vi "dfd_FIR Linear Phase Validation.vi"(8 "error in (no error)":errorcluster, 11 "H(n) in":dbl[](array[numeric])) -> (0 "error out":errorcluster, 3 "H(n) out":dbl[](array[numeric]))   [LabVIEW 2017, in "NI_DigFilter_Design.lvlib"]
uses:
  <vilib>/addons/Digital Filter Design/NI_DigFilter_Design.lvlib
  <vilib>/addons/Digital Filter Design/_Misc.llb/dfd_X Equal Y (Array).vi
  <vilib>/addons/Digital Filter Design/_Misc.llb/dfd_Error Handlers (Single).vi
  <vilib>/addons/Digital Filter Design/NI_DigFilterLicensed.lvlib
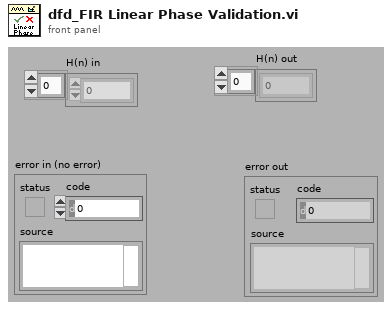
[diagram p1: front panel]
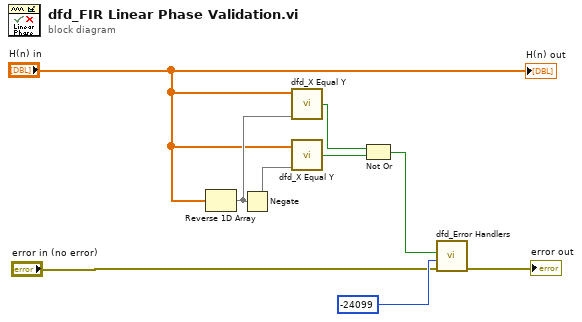
[diagram p0: block diagram]
diagram:
  n1 = Reverse 1D Array(array="H(n) in") -> (reversed array=w5:dbl[])
  n2 = Negate(x=w5) -> (-x=w3:dbl[])
  n3 = call-poly <vilib>:"dfd_X Equal Y.vi"("x"="H(n) in", "y"=w5) -> ("x = y?"=w1:bool)  [unwired: 1 in, 4 out]
  n4 = call-poly <vilib>:"dfd_X Equal Y.vi"("x"="H(n) in", "y"=w3) -> ("x = y?"=w2:bool)  [unwired: 1 in, 4 out]
  n5 = Not Or(1:w2, 2:w1) -> (0:w6:bool)
  n6 = call-poly <vilib>:"dfd_Error Handlers.vi"("error in (no error)"="error in (no error)", "error code"=-24099 ("ERR_NOT_LINEAR_PHASE_FIR"), "condition failed?"=w6) -> ("error out"=→"error out":errorcluster)  [unwired: 8 out]
  "H(n) out" <- "H(n) in"
